vi "Show Items.vi"(8 "error in":errorcluster, 10 "Item Tags":string[](array[string]), 11 "TreeControl in":refnum<vi>) -> (0 "error out":errorcluster)   [LabVIEW 2013, in "LVTM.lvlib"]
uses:
  LVTM.lvlib
  <vilib>/Utility/miscctls.llb/LVNodeAndColumnTypeDef.ctl
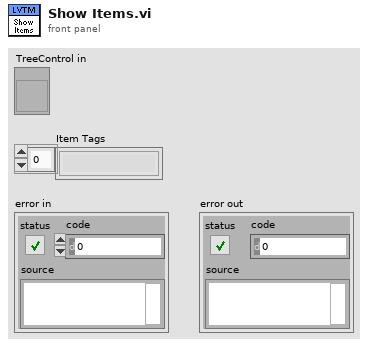
[diagram p1: front panel]
types:
  T1 = typedef "LVNodeAndColumnTypeDef.ctl" = cluster{"Node":string, "Column":i32}
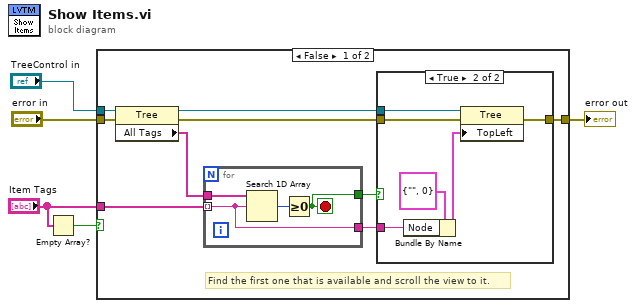
[diagram p0: block diagram]
diagram:
  n1 = Empty Array?(array="Item Tags") -> (empty?=w1:bool)
  n2 = case shown="False" w1 {
    tunnel: "error in" -> [w14 w26]
    tunnel: "TreeControl in" -> [w12 _]
    tunnel: [w7 w26] -> w3
    tunnel: "Item Tags" -> [w6 _]
    frame False {
      # "Find the first one that is available and scroll the view to it."
      n3 = property class="Tree"(reference=w12, error in=w14) -> (reference out=w8:refnum<vi>, error out=w9:errorcluster, "All Tags"=w13:string[])
      n4 = for {
        tunnel: w6 -> [w23] mode=indexing
        tunnel: w13 -> [w25]
        tunnel: [w23] -> w10
        tunnel: [w22] -> w11
        stop <- w22 stop-if-true
        n5 = Search 1D Array(1D array=w25, element=w23) -> (index of element=w24:i32)  [unwired: 1 in]
        n6 = Greater Or Equal To 0?(x=w24) -> (x >= 0?=w22:bool)
      }
      n7 = case shown="True" w11 {
        tunnel: w10 -> [_ w17]
        tunnel: w9 -> [w15 w21]
        tunnel: w8 -> [_ w20]
        tunnel: [w15 w16] -> w7
        frame False {
        }
        frame True {
          n8 = Bundle By Name(cluster=T1 {"Node"="", "Column"=0} ("Top Left Visible Cell"), "Node"=w17) -> (w18:T1)
          n9 = property class="Tree"(reference=w20, error in=w21, "TopLeft"=w18) -> (error out=w16:errorcluster)  [unwired: 1 out]
        }
      }
    }
    frame True {
    }
  }
  "error out" <- w3
